vi "Part 1.vi"(11 "Input":string) -> (3 "Output":i32)   [LabVIEW 2021]
panel:
  out "Waveform Graph":i32[](graph)
  out "min index(es)":i32
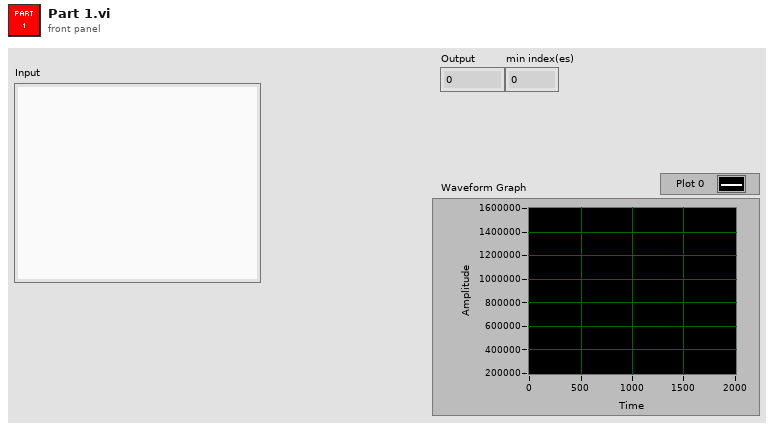
[diagram p1: front panel]
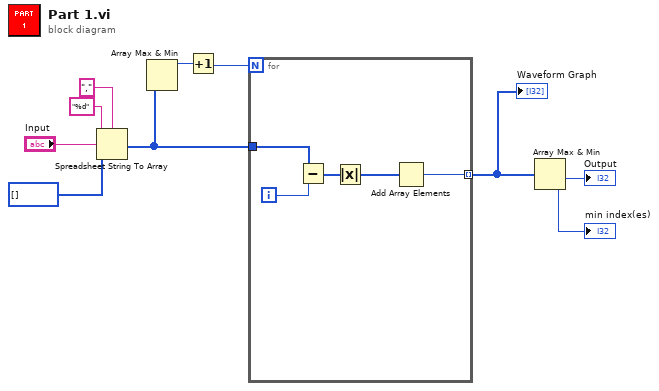
[diagram p0: block diagram]
diagram:
  n1 = Spreadsheet String To Array(delimiter (Tab)=",", format string="%d", spreadsheet string="Input", array type (2D Dbl)=i32[] []) -> (array=w5:i32[])
  n2 = Array Max & Min(array=w5) -> (max value=w4:i32)  [unwired: 3 out]
  n3 = Increment(x=w4) -> (x+1=w3:i32)
  n4 = for {
    N: w3 -> [_]
    tunnel: w5 -> [w14]
    tunnel: [w11] -> w1 mode=indexing
    i -> [w15]
    n5 = Subtract(x=w14, y=w15) -> (x-y=w13:i32[])
    n6 = Absolute Value(x=w13) -> (abs(x)=w12:i32[])
    n7 = Add Array Elements(numeric array=w12) -> (sum=w11:i32)
  }
  "Waveform Graph" <- w1
  n8 = Array Max & Min(array=w1) -> (min value=→"Output":i32, min index (indices)=→"min index(es)":i32)  [unwired: 2 out]
